vi "Read Digital Inputs.vi"() -> ()   [LabVIEW 2020]
panel:
  in  "stop":bool
  out "Numeric":dbl
  out "Array":bool[](array[boolean])
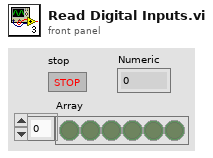
[diagram p1: front panel]
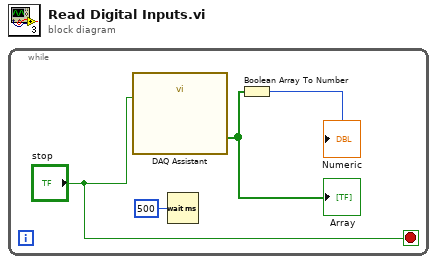
[diagram p0: block diagram]
diagram:
  n1 = while {
    stop <- "stop" stop-if-true
    n2 = call "DAQ Assistant"("stop (T)"="stop") -> ("data"=w2:bool[])  [unwired: 16 in, 2 out]
    "Array" <- w2
    n3 = Wait (ms)(milliseconds to wait=u32 500) -> ()  [unwired: 1 out]
    n4 = Boolean Array To Number(Boolean array=w2) -> (number=→"Numeric":u32)
  }
